vi "Inst.RP100.setState.vi"(8 "error in (no error)":errorcluster, 10 "data in":variant, 11 "Inst.RP100 in":refnum<class "Inst.RP100.lvclass">) -> (0 "error out":errorcluster, 3 "Inst.RP100 out":refnum<class "Inst.RP100.lvclass">)   [LabVIEW 2019, in "Inst.RP100.lvclass"]
uses:
  Inst.RP100.lvclass
  Typedefs/Output Channel--Enum.ctl
  Typedefs/setOutput--Cluster.ctl
  Typedefs/Output State--Enum.ctl
  Inst.RP100.lvclass/Inst.RP100.ctl
  bc4c31a2-e180-42ef-bc87-c6c1dd52d23b.vi
  <vilib>/JDP Science/JSONtext/JSON text to Variant.vi
  <vilib>/JDP Science/JSONtext/LVClass Serializer/JSONtext LVClass Serializer.lvclass
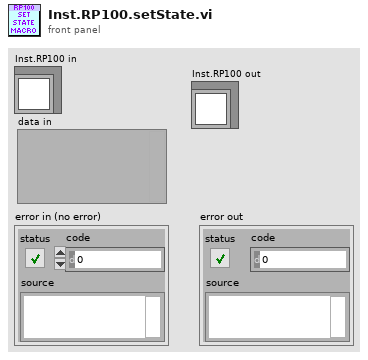
[diagram p1: front panel]
types:
  T1 = typedef "Inst.RP100.lvclass/setOutput--Cluster.ctl" = cluster{"State":T2}
  T2 = typedef "Inst.RP100.lvclass/Output State--Enum.ctl" = enum16{"Shorted", "Enabled"}
  T3 = typedef "Inst.RP100.lvclass/Output Channel--Enum.ctl" = enum16{"Output 1", "Output 2"}
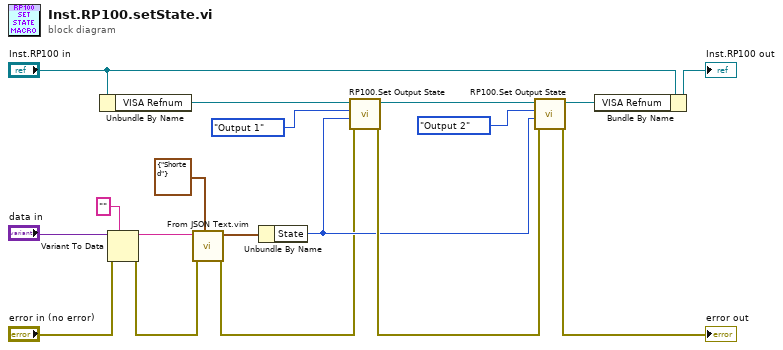
[diagram p0: block diagram]
diagram:
  n1 = Unbundle By Name("Inst.RP100 in") -> ("VISA Refnum"=w12:refnum<visa-resource-name>)
  n2 = Variant To Data(error in="error in (no error)", type="", Variant="data in") -> (data=w5:string, error out=w1:errorcluster)
  n3 = call "From JSON Text.vim"("Data Type and Default Value"=T1 {"State"=enum."Shorted"} ("Data out"), "error in (no error)"=w1, "JSON"=w5) -> ("error out"=w4:errorcluster, "Data out"=w3:T1)  [unwired: 7 in]
  n4 = Unbundle By Name(w3) -> ("State"=w13:T2)
  n5 = call "RP100.Set Output State.vi"("error in (no error)"=w4, "Output State"=w13, "Output Channel"=Output_Channel--Enum."Output 1", "VISA resource name"=w12) -> ("error out"=w17:errorcluster, "VISA Refnum out"=w16:refnum<visa-resource-name>)  [unwired: 5 in, 1 out]
  n6 = call "RP100.Set Output State.vi"("error in (no error)"=w17, "Output State"=w13, "Output Channel"=Output_Channel--Enum."Output 2", "VISA resource name"=w16) -> ("error out"=→"error out":errorcluster, "VISA Refnum out"=w11:refnum<visa-resource-name>)  [unwired: 5 in, 1 out]
  n7 = Bundle By Name(cluster="Inst.RP100 in", "VISA Refnum"=w11) -> (→"Inst.RP100 out":refnum<class "Inst.RP100.lvclass">)
